vi "1 channel coutinous samples.vi"() -> ()   [LabVIEW 2020]
panel:
  in  "stop (F)":bool
  in  "rate":dbl=1000.0
  in  "number of samples":i32=100
  out "Waveform Chart":dynamicdata(graph)
  out "Waveform Graph":dynamicdata(graph)
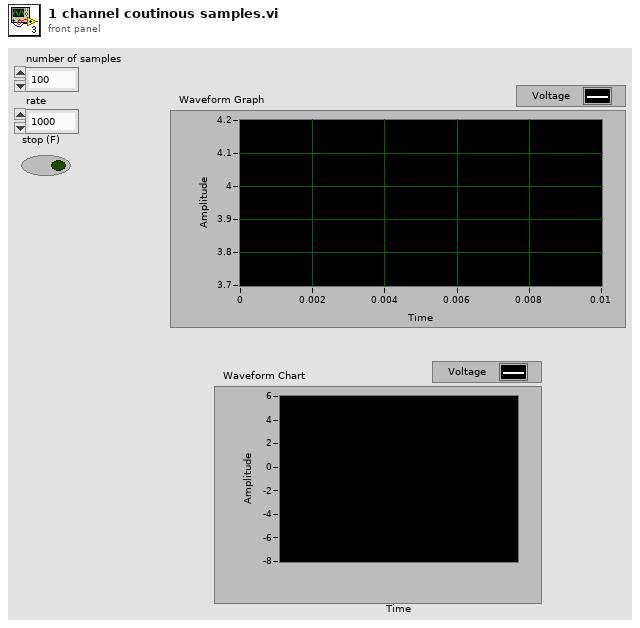
[diagram p1: front panel]
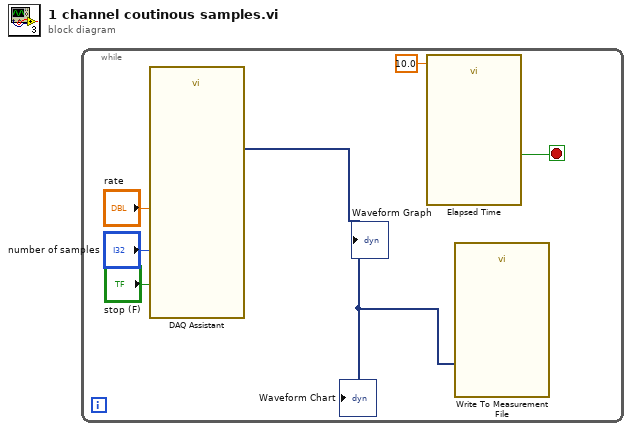
[diagram p0: block diagram]
diagram:
  n1 = while {
    stop <- w3 stop-if-true
    n2 = call "DAQ Assistant"("rate"="rate", "number of samples"="number of samples", "stop (F)"="stop (F)") -> ("data"=w1:dynamicdata)  [unwired: 13 in, 3 out]
    "Waveform Graph" <- w1
    "Waveform Chart" <- w1
    n3 = call "Elapsed Time"("Time Target (s)"=10.0) -> ("Time has Elapsed"=w3:bool)  [unwired: 11 in, 7 out]
    n4 = call "Write To Measurement File"("Signals"=w1) -> ()  [unwired: 16 in, 3 out]
  }
